vi "TDMSwritedata.vi"() -> ()   [LabVIEW 2018, in "RW_Protocols.lvlib"]
uses:
  RW_Protocols.lvlib
panel:
  out "Waveform Graph":dynamicdata(graph)
  in  "file path":path=path "D:/Data/Mai/test target/waveformtest"
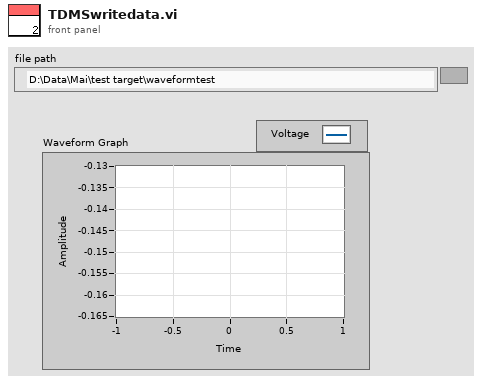
[diagram p1: front panel]
types:
  T1 = enum16{"open", "open or create", "create or replace", "create", "open (read-only)"}
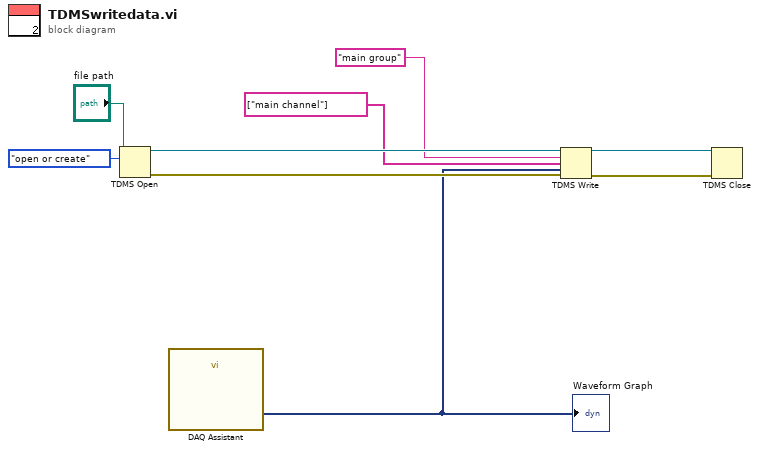
[diagram p0: block diagram]
diagram:
  n1 = TDMS Open(10:T1."open or create" ("operation (0:open)"), 11:"file path") -> (0:w4:errorcluster, 3:w7:refnum<k34>)  [unwired: 5 in]
  n2 = call "DAQ Assistant"() -> ("data"=w1:dynamicdata)  [unwired: 17 in, 2 out]
  "Waveform Graph" <- w1
  n3 = TDMS Write(0:w7, 5:"main group" ("group name in (Untitled)"), 7:string[] ["main channel"] ("channel name(s) in (Untitled)"), 9:w1, 11:w4) -> (4:w6:refnum<k34>, 15:w5:errorcluster)  [unwired: 1 in, 2 out]
  n4 = TDMS Close(8:w5, 11:w6) -> ()  [unwired: 2 out]
